vi "Data(String to Data).vi"(10 "当前状态":string, 11 "数据":waveform(sgl)[](array[waveform])) -> (3 "数组":waveform(sgl)[](array[waveform]))   [LabVIEW 2020, in "人体健康监测系统.lvclass"]
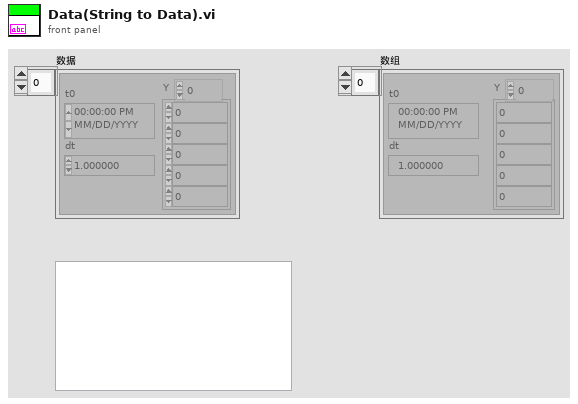
[diagram p1: front panel]
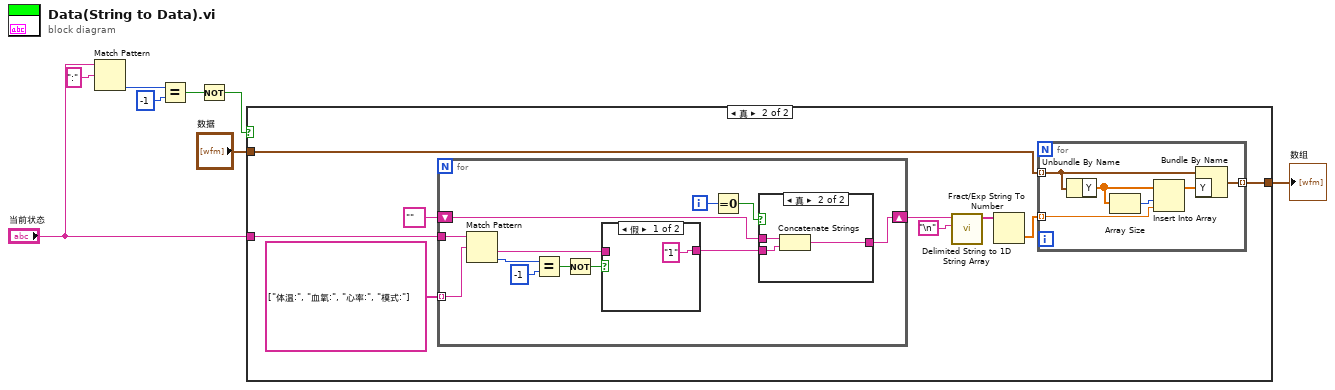
[diagram p0: block diagram]
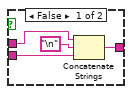
[diagram p3: hidden frame]
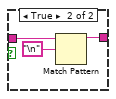
[diagram p4: hidden frame]
diagram:
  n1 = Match Pattern(string="当前状态", regular expression=":" ("正则表达式")) -> (offset past match=w7:i32)  [unwired: 1 in, 3 out]
  n2 = Equal?(x=w7, y=-1) -> (x = y?=w6:bool)
  n3 = Not(x=w6) -> (.not. x?=w3:bool)
  n4 = case shown="真" w3 {
    tunnel: "当前状态" -> [_ w16]
    tunnel: "数据" -> [w9 w12]
    tunnel: [w9 w10] -> w1
    frame False {
    }
    frame True {
      n5 = for {
        tunnel: string[] ["体温:", "血氧:", "心率:", "模式:"] -> [w26] mode=indexing
        tunnel: w16 -> [w36]
        shift-right: [w28] -> w15
        shift-left: "" ("读取缓冲区") -> [w31]
        i -> [w30]
        n6 = Match Pattern(string=w36, regular expression=w26) -> (after substring=w32:string, offset past match=w35:i32)  [unwired: 1 in, 2 out]
        n7 = Equal?(x=w35, y=-1) -> (x = y?=w33:bool)
        n8 = Not(x=w33) -> (.not. x?=w27:bool)
        n9 = case shown="假" w27 {
          tunnel: w32 -> [_ w47]
          tunnel: ["1" ("读取缓冲区") w45] -> w25
          frame False {
          }
          frame True {
            n10 = Match Pattern(string=w47, regular expression="\n") -> (before substring=w45:string)  [unwired: 1 in, 3 out]
          }
        }
        n11 = Equal To 0?(x=w30) -> (x = 0?=w29:bool)
        n12 = case shown="真" w29 {
          tunnel: w31 -> [w40 w43]
          tunnel: w25 -> [w38 w42]
          tunnel: [w37 w41] -> w28
          frame False {
            n13 = Concatenate Strings(w40, "\n", w38) -> (w37:string)
          }
          frame True {
            n14 = Concatenate Strings(w43, w42) -> (w41:string)
          }
        }
      }
      n15 = call <vilib>:"Delimited String to 1D String Array.vi"("delimiter"="\n", "delimited string"=w15) -> ("string array"=w13:string[])  [unwired: 9 in]
      n16 = Fract/Exp String To Number(string=w13) -> (number=w11:dbl[])  [unwired: 3 in, 1 out]
      n17 = for {
        tunnel: w12 -> [w24] mode=indexing
        tunnel: w11 -> [w23] mode=indexing
        tunnel: [w19] -> w10 mode=indexing
        n18 = Unbundle By Name(w24) -> ("Y"=w22:sgl[])
        n19 = Array Size(array=w22) -> (size(s)=w21:i32)
        n20 = Insert Into Array(array=w22, index=w21, new element=w23) -> (w20:sgl[])
        n21 = Bundle By Name(cluster=w24, "Y"=w20) -> (w19:waveform(sgl))
      }
    }
  }
  "数组" <- w1
